vi "Choose Active API.vi"(7 "Host Resources":T10, 11 "Hardware Configuration in":T1) -> (3 "Hardware Configuration out":T1)   [LabVIEW 2021, in "Acquisition.lvlib"]
doc: "Choose the best API for the measurements according to 'Hardware Configuration in' and 'Host Resources'.\n\nIf either driver APIs or DAQ devices cannot be found on the host, choose the Simulated API."
uses:
  Acquisition.lvlib
  Hardware Configuration.ctl
  Channel Settings.ctl
  IO Device.ctl
  Sensor Type.ctl
  Interval Timer/Repeat Interval.ctl
  Interval Timer/Interval Length.ctl
  Interval Timer/Interval Token.ctl
  IO Context.ctl
  IO API.ctl
  Host Resources.ctl
  Host Software Package.ctl
  Host IO Resource.ctl
  Interval Timer/Interval Timer.lvlib
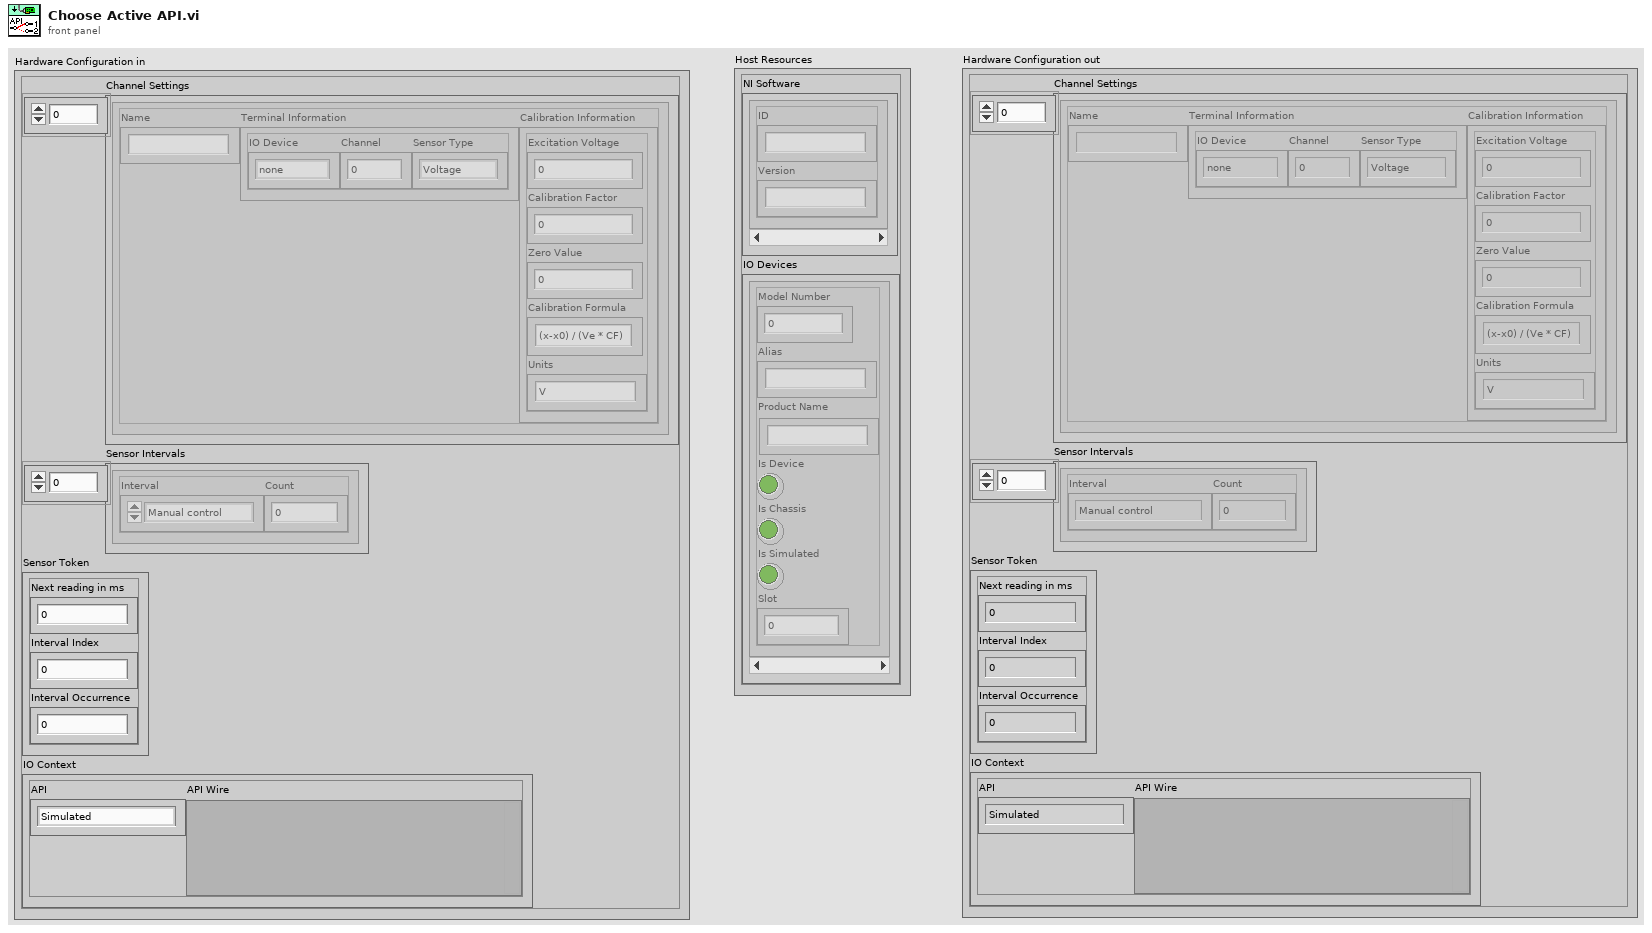
[diagram p1: front panel]
types:
  T1 = typedef "Acquisition.lvlib/Hardware Configuration.ctl" = cluster{"Channel Settings":T2[], "Sensor Intervals":T5[], "Sensor Token":T7, "IO Context":T8}
  T2 = typedef "Acquisition.lvlib/Channel Settings.ctl" = cluster{"Name":string, "Terminal Information":cluster{"IO Device":T3, "Channel":i32, "Sensor Type":T4}, "Calibration Information":cluster{"Excitation Voltage":dbl, "Calibration Factor":dbl, "Zero Value":dbl, "Calibration Formula":string, "Units":string}}
  T3 = typedef "Acquisition.lvlib/IO Device.ctl" = enum16{"none", "9219", "9401"}
  T4 = typedef "Acquisition.lvlib/Sensor Type.ctl" = enum16{"Voltage", "Load", "Pressure", "Encoder"}
  T5 = typedef "Interval Timer.lvlib/Repeat Interval.ctl" = cluster{"Interval":T6, "Count":i32}
  T6 = typedef "Interval Timer.lvlib/Interval Length.ctl" = enum16{"Manual control", "1 second", "10 seconds", "30 seconds", "60 seconds", "600 seconds", "1200 seconds", "3600 seconds"}
  T7 = typedef "Interval Timer.lvlib/Interval Token.ctl" = cluster{"Next reading in ms":u32, "Interval Index":i32, "Interval Occurrence":i32}
  T8 = typedef "Acquisition.lvlib/IO Context.ctl" = cluster{"API":T9, "API Wire":variant}
  T9 = typedef "Acquisition.lvlib/IO API.ctl" = enum16{"Simulated", "DAQmx"}
  T10 = typedef "Acquisition.lvlib/Host Resources.ctl" = cluster{"NI Software":T11[], "IO Devices":T12[]}
  T11 = typedef "Acquisition.lvlib/Host Software Package.ctl" = cluster{"ID":string, "Version":string}
  T12 = typedef "Acquisition.lvlib/Host IO Resource.ctl" = cluster{"Model Number":u32, "Alias":string, "Product Name":string, "Is Device":bool, "Is Chassis":bool, "Is Simulated":bool, "Slot":i32}
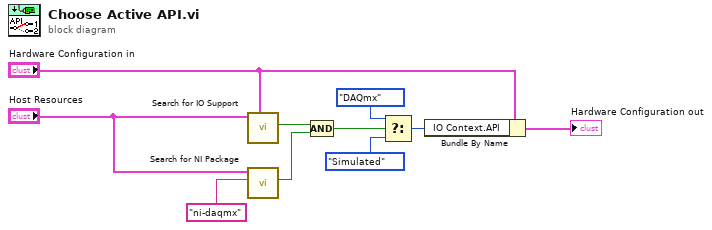
[diagram p0: block diagram]
diagram:
  n1 = call "Search for IO Support.vi"("Hardware Configuration"="Hardware Configuration in", "Host Resources"="Host Resources") -> ("IO supports configuration?"=w9:bool)  [unwired: 9 in]
  n2 = call "Search for NI Package.vi"("software package ID"="ni-daqmx", "Host Resources"="Host Resources") -> ("Is package installed?"=w10:bool)  [unwired: 9 in]
  n3 = Compound Arithmetic op=AND(w9, w10) -> (w6:bool)
  n4 = Select(t=IO_API."DAQmx" ("API"), s=w6, f=IO_API."Simulated" ("API")) -> (s? t:f=w4:T9)
  n5 = Bundle By Name(cluster="Hardware Configuration in", "IO Context.API"=w4) -> (→"Hardware Configuration out":T1)
